vi "ChoreoToBordeauxCoordinates.vi"(10 "Choreo Type":T3(array[cluster])) -> (2 "Bordeaux Type":T5, 3 "Trajectory Data":T2(array[cluster]), 5 "Points out":T4[](array[typedef]))   [LabVIEW 2025]
uses:
  swerve-template/Type Definitions/Data/Robot Velocities.ctl
  Types/Segment Type.ctl
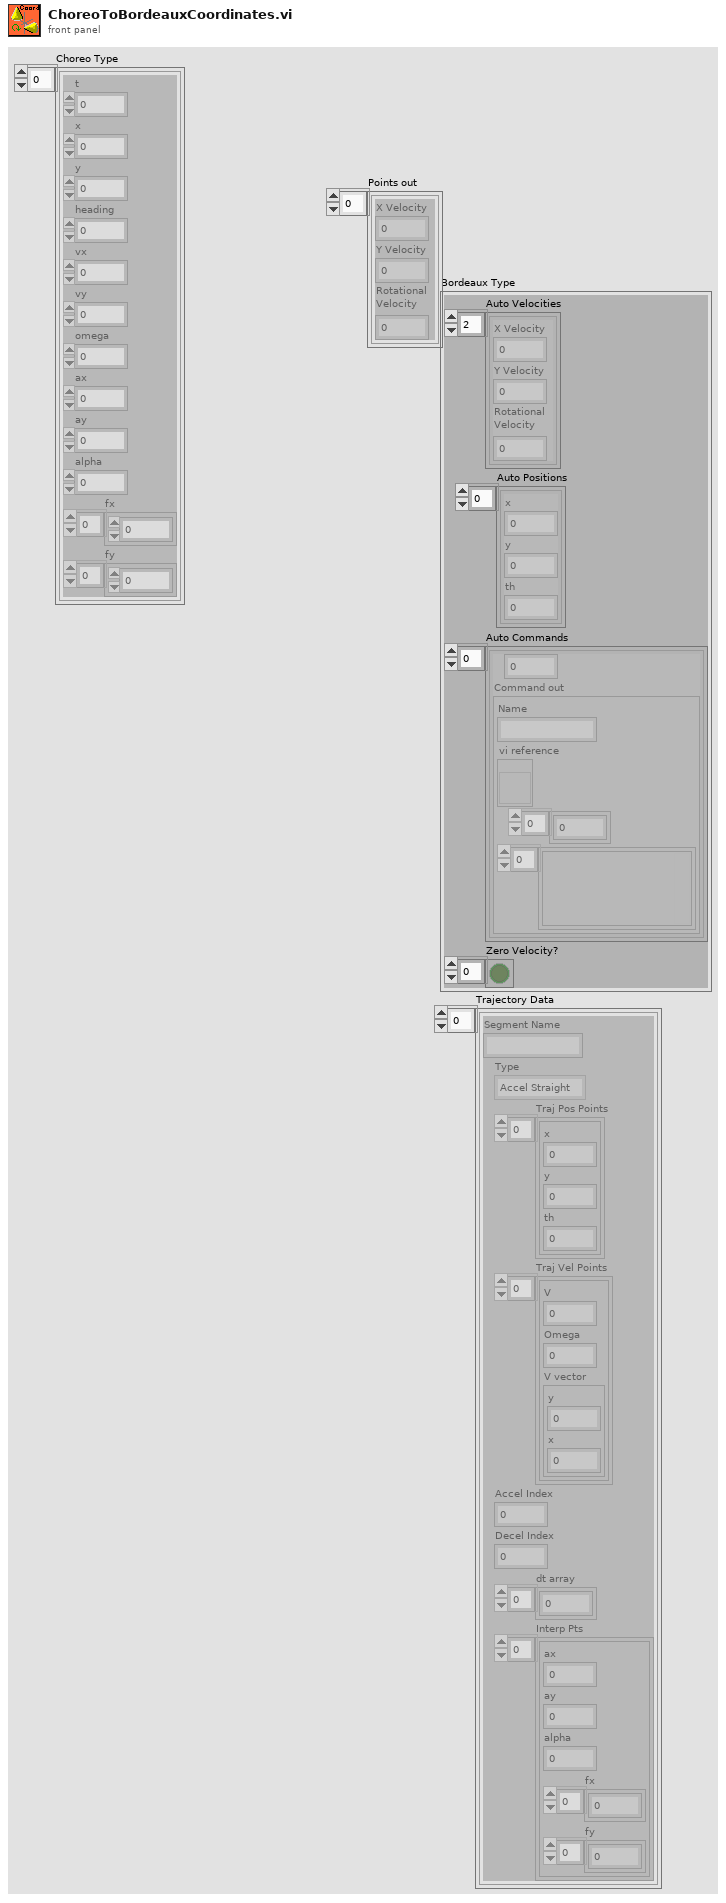
[diagram p1: front panel]
types:
  T1 = typedef "Segment Type.ctl" = enum16{"Accel Straight", "Const Straight", "Blend", "Circle", "Bezier", "Choreo"}
  T2 = cluster{"Segment Name":string, "Type":T1, "Traj Pos Points":cluster{"x":dbl, "y":dbl, "th":dbl}[], "Traj Vel Points":cluster{"V":dbl, "Omega":dbl, "V vector":cluster{"y":dbl, "x":dbl}}[], "Accel Index":i32, "Decel Index":i32, "dt array":dbl[], "Interp Pts":cluster{"ax":dbl, "ay":dbl, "alpha":dbl, "fx":dbl[], "fy":dbl[]}[]}[]
  T3 = cluster{"t":dbl, "x":dbl, "y":dbl, "heading":dbl, "vx":dbl, "vy":dbl, "omega":dbl, "ax":dbl, "ay":dbl, "alpha":dbl, "fx":dbl[], "fy":dbl[]}[]
  T4 = typedef "Robot Velocities.ctl" = cluster{"X Velocity":dbl, "Y Velocity":dbl, "Rotational \nVelocity":dbl}
  T5 = cluster{"Auto Velocities":T4[], "Auto Positions":cluster{"x":dbl, "y":dbl, "th":dbl}[], "Auto Commands":cluster{dbl, "Command out":cluster{"Name":string, "vi reference":refnum<vi>, i32[], variant[]}}[], "Zero Velocity?":bool[]}
  T6 = cluster{"Segment Name":string, "Type":T1, "Traj Pos Points":cluster{"x":dbl, "y":dbl, "th":dbl}[], "Traj Vel Points":cluster{"V":dbl, "Omega":dbl, "V vector":cluster{"y":dbl, "x":dbl}}[], "Accel Index":i32, "Decel Index":i32, "dt array":dbl[], "Interp Pts":cluster{"ax":dbl, "ay":dbl, "alpha":dbl, "fx":dbl[], "fy":dbl[]}[]}
  T7 = cluster{dbl, "Command out":cluster{"Name":string, "vi reference":refnum<vi>, i32[], variant[]}}[]
  T8 = cluster{"ax":dbl, "ay":dbl, "alpha":dbl, "fx":dbl[], "fy":dbl[]}
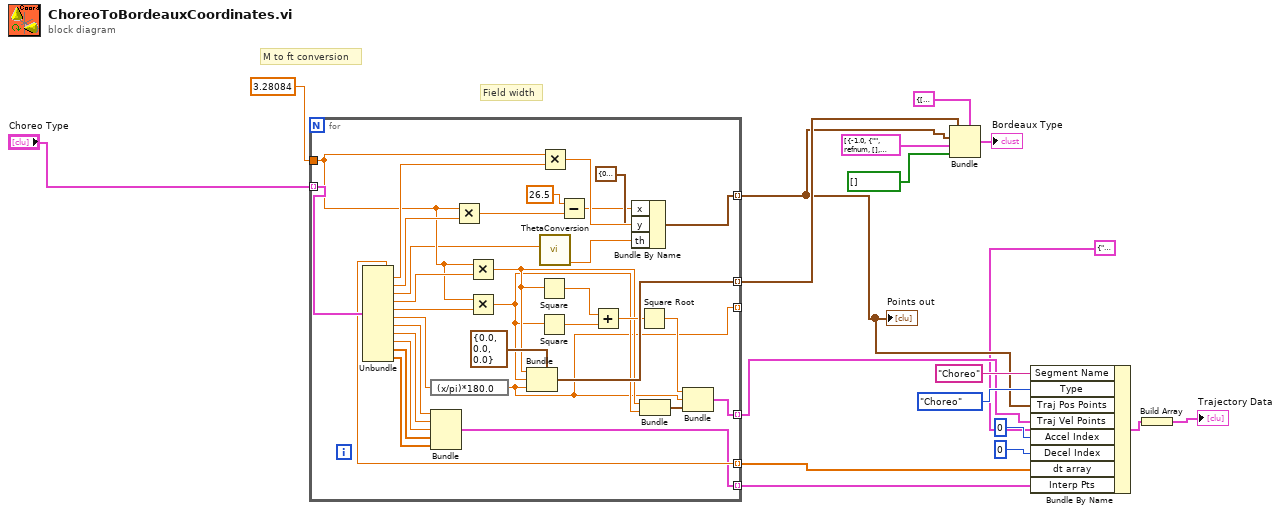
[diagram p0: block diagram]
diagram:
  # "M to ft conversion"
  # "Field width"
  n1 = for {
    tunnel: "Choreo Type" -> [w51] mode=indexing
    tunnel: 3.28084 -> [w31]
    tunnel: [w48] -> w6 mode=indexing
    tunnel: [w47] -> w13 mode=indexing
    tunnel: [w35] -> w7 mode=indexing
    tunnel: [w28] -> _ mode=indexing
    tunnel: [w25] -> w3 mode=indexing
    tunnel: [w19] -> w2 mode=indexing
    n2 = Unbundle(w51) -> ("t"=w25:dbl, "x"=w41:dbl, "y"=w50:dbl, "heading"=w27:dbl, "vx"=w34:dbl, "vy"=w32:dbl, "omega"=w29:dbl, "ax"=w24:dbl, "ay"=w23:dbl, "alpha"=w22:dbl, "fx"=w21:dbl[], "fy"=w20:dbl[])
    n3 = expression code="(x/pi)*180.0" ("radians to degrees")(w29) -> (w28:dbl)
    n4 = Bundle("ax"=w24, "ay"=w23, "alpha"=w22, "fx"=w21, "fy"=w20) -> (w19:T8)  [unwired: 1 in]
    n5 = Multiply(x=w31, y=w50) -> (x*y=w43:dbl)
    n6 = Multiply(x=w31, y=w34) -> (x*y=w33:dbl)
    n7 = Multiply(x=w31, y=w32) -> (x*y=w30:dbl)
    n8 = Bundle(cluster=T4 {"X Velocity"=0.0, "Y Velocity"=0.0, "Rotational \nVelocity"=0.0} ("Robot Velocities"), "X Velocity"=w33, "Y Velocity"=w30, "Rotational \nVelocity"=w28) -> (w47:T4)
    n9 = Square(x=w33) -> (x^2=w40:dbl)
    n10 = Square(x=w30) -> (x^2=w39:dbl)
    n11 = Multiply(x=w31, y=w41) -> (x*y=w49:dbl)
    n12 = call "ThetaConversion.vi"("Input rad"=w27) -> ("out new"=w26:dbl)  [unwired: 10 in]
    n13 = Subtract(x=26.5, y=w43) -> (x-y=w42:dbl)
    n14 = Add(x=w40, y=w39) -> (x+y=w38:dbl)
    n15 = Bundle By Name(cluster=cluster{"x":dbl, "y":dbl, "th":dbl} {"x"=0.0, "y"=0.0, "th"=0.0} ("Cluster"), "x"=w42, "y"=w49, "th"=w26) -> (w48:cluster{"x":dbl, "y":dbl, "th":dbl})
    n16 = Square Root(x=w38) -> (sqrt(x)=w37:dbl)
    n17 = Bundle(w33, w30) -> (w36:cluster{dbl, dbl})  [unwired: 1 in]
    n18 = Bundle(w37, "omega"=w28, w36) -> (w35:cluster{dbl, "omega":dbl, cluster{dbl, dbl}})  [unwired: 1 in]
  }
  "Points out" <- w6
  n19 = Bundle(cluster=T5 {"Auto Velocities"=[], "Auto Positions"=[], "Auto Commands"=[], "Zero Velocity?"=[]} ("Auto Data"), "Auto Velocities"=w13, "Auto Positions"=w6, "Auto Commands"=T7 [{-1.0, "Command out"={"Name"="", "vi reference"=refnum, [], []}}], "Zero Velocity?"=bool[] []) -> (→"Bordeaux Type":T5)
  n20 = Bundle By Name(cluster=T6 {"Segment Name"="", "Type"=enum."Accel Straight", "Traj Pos Points"=[], "Traj Vel Points"=[], "Accel Index"=0, "Decel Index"=0, "dt array"=[], "Interp Pts"=[]}, "Segment Name"="Choreo", "Type"=Segment_Type."Choreo", "Traj Pos Points"=w6, "Traj Vel Points"=w7, "Accel Index"=0, "Decel Index"=0, "dt array"=w3, "Interp Pts"=w2) -> (w12:T6)
  n21 = Build Array(w12) -> (→"Trajectory Data":T2)
